vi "profile_time_simple.vi"(7 "Motor Adress":T1(ring)=enum."3", 8 "error in (no error)":errorcluster, 10 "steps in":i32, 11 "VISA ressource in":refnum<visa-resource-name>="COM7") -> (0 "error out":errorcluster={"status"=FALSE, "code"=1073676294, "source"="VISA Read in write_read.vi"}, 1 "profile time (in ms)":u32, 2 "direction":i32, 3 "VISA ressource out":refnum<visa-resource-name>, 5 "steps":u32)   [LabVIEW 2013]
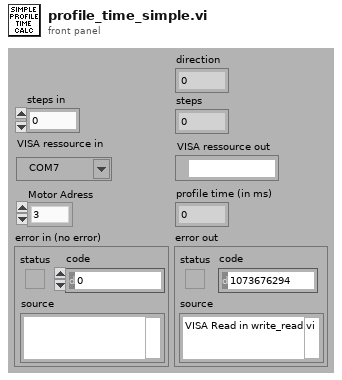
[diagram p1: front panel]
types:
  T1 = enum16{"All", "1", "2", "3", "4", "5", "6", "7", "8"}
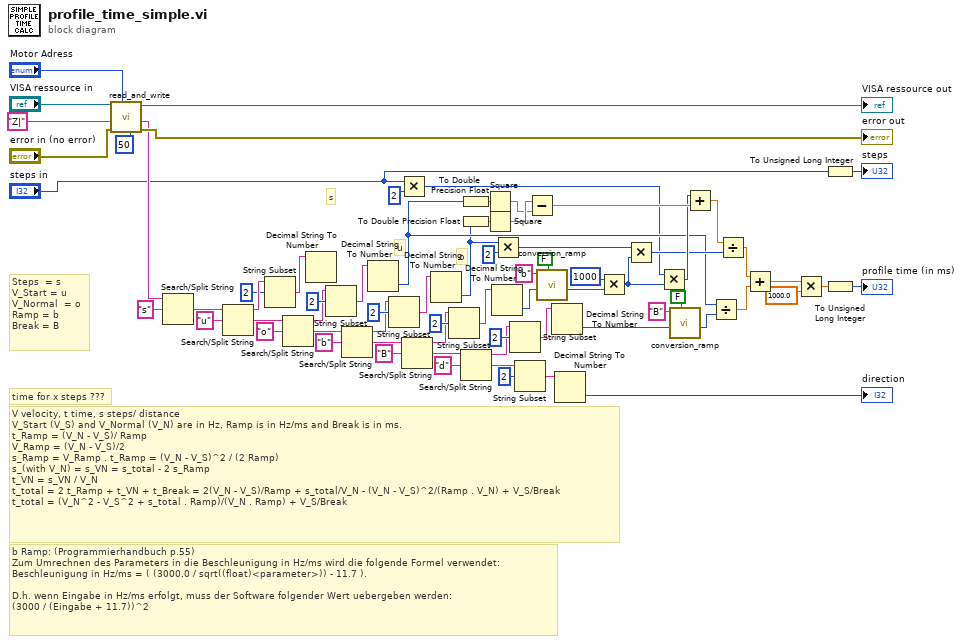
[diagram p0: block diagram]
diagram:
  # "o"
  # "u"
  # "s"
  # "b Ramp: (Programmierhandbuch p.55)\nZum Umrechnen des Parameters in die Beschleunigung in Hz/ms wird die folgende Formel verwendet:\nBeschleunigung in Hz/ms = ( (3000.0 / sqrt((float)<parameter>)) - 11.7 ).\n\nD.h. wenn Eingabe in Hz/ms erfolgt, muss der Software folgender Wert uebergeben werden:\n(3000 / (Eingabe + 11.7))^2"
  # "V velocity, t time, s steps/ distance\nV_Start (V_S) and V_Normal (V_N) are in Hz, Ramp is in Hz/ms and Break is in ms.\nt_Ramp = (V_N - V_S)/ Ramp\nV_Ramp = (V_N - V_S)/2\ns_Ramp = V_Ramp . t_Ramp = (V_N - V_S)^2 / (2 Ramp)\ns_(with V_N) = s_VN = s_total - 2 s_Ramp\nt_VN = s_VN / V_N\nt_total = 2 t_Ramp + t_VN + t_Break = 2(V_N - V_S)/Ramp + s_total/V_N - (V_N - V_S)^2/(Ramp . V_N) + V_S/Break\nt_total = (V_N^2 - V_S^2 + s_total . Ramp)/(V_N . Ramp) + V_S/Break"
  # "time for x steps ???"
  # "Steps  = s\nV_Start = u \nV_Normal  = o\nRamp = b\nBreak = B"
  n1 = call "read_and_write.vi"("additional waiting time"=u32 50, "Motor Adress"="Motor Adress", "error in (no error)"="error in (no error)", "Command"="Z|", "VISA ressource in"="VISA ressource in") -> ("error out"=→"error out":errorcluster, "Answer"=w67:string, "VISA ressource out"=→"VISA ressource out":refnum<visa-resource-name>)  [unwired: 3 in, 1 out]
  n2 = Search/Split String(string=w67, search string/char (-)="s") -> (match + rest of string=w61:string)  [unwired: 1 in, 2 out]
  n3 = Search/Split String(string=w61, search string/char (-)="u") -> (substring before match=w55:string, match + rest of string=w60:string)  [unwired: 1 in, 1 out]
  n4 = String Subset(string=w55, offset (0)=2) -> (substring=w43:string)  [unwired: 1 in]
  n5 = Search/Split String(string=w60, search string/char (-)="o") -> (substring before match=w47:string, match + rest of string=w59:string)  [unwired: 1 in, 1 out]
  n6 = Decimal String To Number(string=w43) -> ()  [unwired: 2 in, 2 out]
  n7 = String Subset(string=w47, offset (0)=2) -> (substring=w42:string)  [unwired: 1 in]
  n8 = Search/Split String(string=w59, search string/char (-)="b") -> (substring before match=w46:string, match + rest of string=w58:string)  [unwired: 1 in, 1 out]
  n9 = Decimal String To Number(string=w42) -> (number=w17:i32)  [unwired: 2 in, 1 out]
  n10 = String Subset(string=w46, offset (0)=2) -> (substring=w41:string)  [unwired: 1 in]
  n11 = Multiply(x="steps in", y=2) -> (x*y=w12:i32)
  n12 = Search/Split String(string=w58, search string/char (-)="B") -> (substring before match=w45:string, match + rest of string=w56:string)  [unwired: 1 in, 1 out]
  n13 = Decimal String To Number(string=w41) -> (number=w11:i32)  [unwired: 2 in, 1 out]
  n14 = String Subset(string=w45, offset (0)=2) -> (substring=w40:string)  [unwired: 1 in]
  n15 = To Double Precision Float(number=w17) -> (double precision float=w5:dbl)
  n16 = To Double Precision Float(number=w11) -> (double precision float=w4:dbl)
  n17 = Search/Split String(string=w56, search string/char (-)="d") -> (substring before match=w44:string, match + rest of string=w21:string)  [unwired: 1 in, 1 out]
  n18 = Square(x=w5) -> (x^2=w31:dbl)
  n19 = Square(x=w4) -> (x^2=w32:dbl)
  n20 = Decimal String To Number(string=w40) -> (number=w35:i32)  [unwired: 2 in, 1 out]
  n21 = Multiply(x=w11, y=2) -> (x*y=w9:i32)
  n22 = String Subset(string=w44, offset (0)=2) -> (substring=w39:string)  [unwired: 1 in]
  n23 = String Subset(string=w21, offset (0)=2) -> (substring=w20:string)  [unwired: 1 in]
  n24 = Subtract(x=w32, y=w31) -> (x-y=w30:dbl)
  n25 = call "conversion_ramp.vi"("From Hz/ms to Driver"=FALSE, "Value"=w35, "Command"="b") -> ("Value out"=w8:i32)  [unwired: 7 in, 1 out]
  n26 = Decimal String To Number(string=w39) -> (number=w23:i32)  [unwired: 2 in, 1 out]
  n27 = Decimal String To Number(string=w20) -> (number=→"direction":i32)  [unwired: 2 in, 1 out]
  n28 = Multiply(x=1000, y=w8) -> (x*y=w6:i32)
  n29 = Multiply(x=w9, y=w6) -> (x*y=w27:i32)
  n30 = Multiply(x=w12, y=w6) -> (x*y=w29:i32)
  n31 = call "conversion_ramp.vi"("From Hz/ms to Driver"=FALSE, "Value"=w23, "Command"="B") -> ("Value out"=w19:i32)  [unwired: 7 in, 1 out]
  n32 = Add(x=w29, y=w30) -> (x+y=w28:dbl)
  n33 = Divide(x=w17, y=w19) -> (x/y=w18:dbl)
  n34 = Divide(x=w28, y=w27) -> (x/y=w26:dbl)
  n35 = Add(x=w26, y=w18) -> (x+y=w16:dbl)
  n36 = Multiply(x=w16, y=1000.0) -> (x*y=w14:dbl)
  n37 = To Unsigned Long Integer(number="steps in") -> (unsigned 32bit integer=→"steps":u32)
  n38 = To Unsigned Long Integer(number=w14) -> (unsigned 32bit integer=→"profile time (in ms)":u32)
